vi "RunTimeMenu_Add_Volt_Chan.vi"(8 "error in (no error)":errorcluster, 11 "Node Ptr":u64 format="%.0x") -> (0 "error out":errorcluster)   [LabVIEW 2018, in "NI PXI-4110 Programmable Power Supply Custom Device.lvlib"]
uses:
  NI PXI-4110 Programmable Power Supply Custom Device.lvlib
  <vilib>/NI VeriStand/Custom Device API/Custom Device API.lvlib
  4110_Global.vi
  <vilib>/NI Veristand/Custom Device API/Get Item Property (U16).vi
panel:
  in  "Tag":string
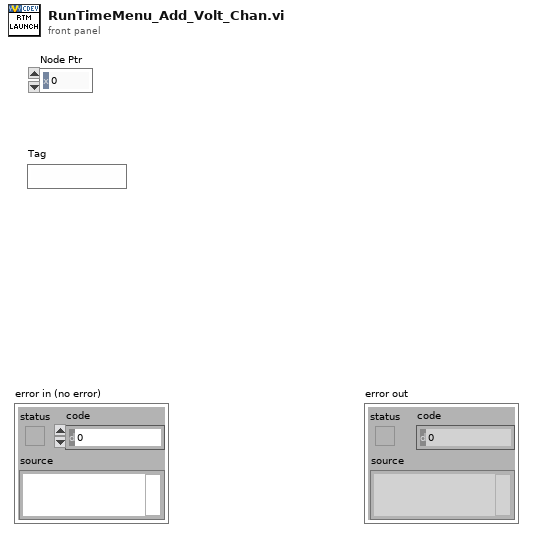
[diagram p1: front panel]
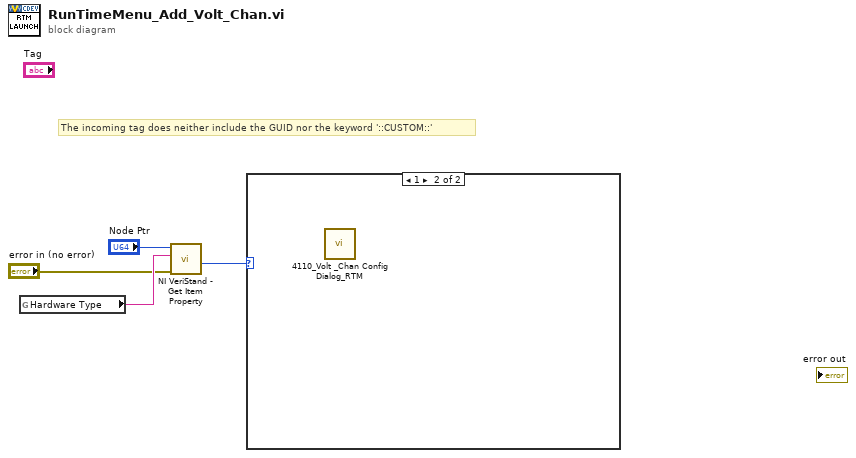
[diagram p0: block diagram]
diagram:
  # "The incoming tag does neither include the GUID nor the keyword '::CUSTOM::'"
  n1 = global read "4110_Global.vi" "Hardware Type"() -> (w3:string)
  n2 = call-poly <vilib>:"NI VeriStand - Get Item Property.vi"("error in (no error)"="error in (no error)", "Property Name"=w3, "Item Ref in"="Node Ptr") -> ("Value"=w1:u16)  [unwired: 5 in, 3 out]
  n3 = case shown="1" w1 {
    frame 0, Default {
    }
    frame 1 {
      n4 = call "4110_Volt _Chan Config Dialog_RTM.vi"() -> ()  [unwired: 6 in, 6 out]
    }
  }
